vi "Update WayPt Angles.vi"(6 "Min R":dbl, 7 "Propagate":bool, 8 "Blends In":T1[](array[typedef]), 9 "Index":i32, 10 "Waypoints in":cluster{"x":dbl, "y":dbl, "th":dbl}[](array[cluster]), 11 "th":dbl) -> (1 "Blends Out":T1[](array[typedef]), 3 "Waypoints out":cluster{"x":dbl, "y":dbl, "th":dbl}[](array[cluster]))   [LabVIEW 2019]
uses:
  BlendType.ctl
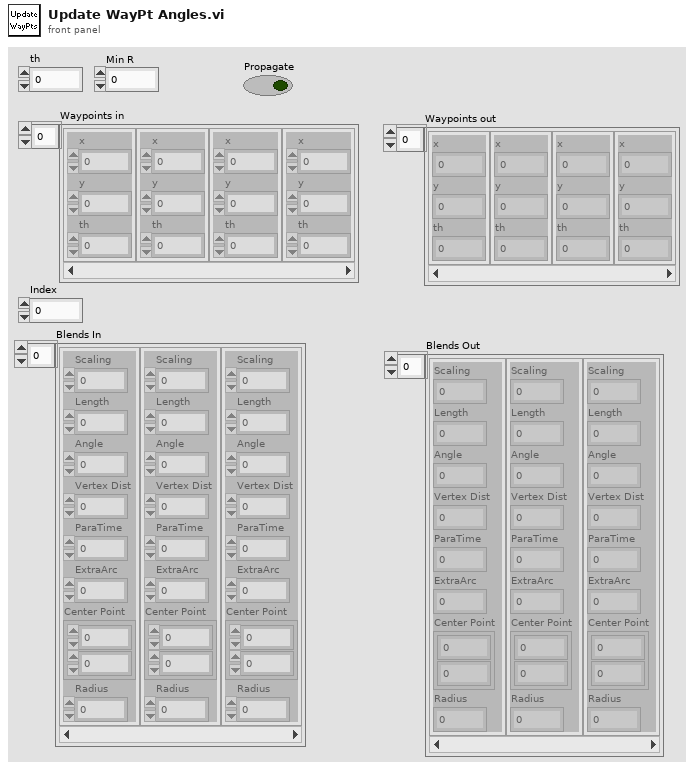
[diagram p1: front panel]
types:
  T1 = typedef "BlendType.ctl" = cluster{"Scaling":dbl, "Length":dbl, "Angle":dbl, "Vertex Dist":dbl, "ParaTime":dbl, "ExtraArc":dbl, "Center Point":cluster{dbl, dbl}, "Radius":dbl}
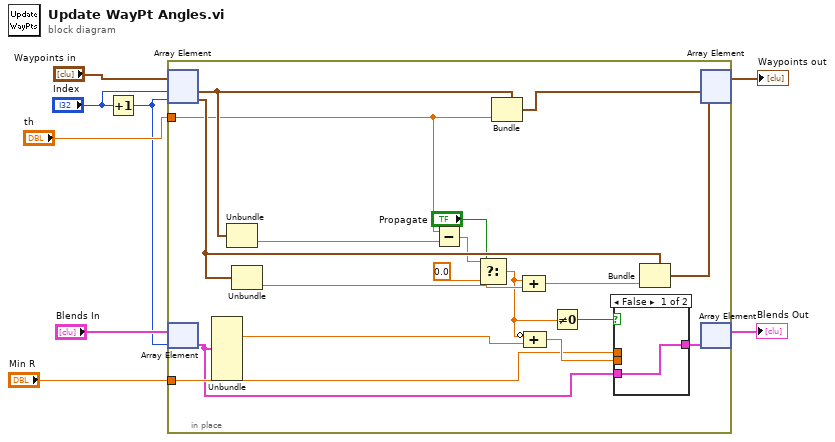
[diagram p0: block diagram]
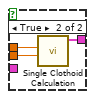
[diagram p2: hidden frame]
diagram:
  n1 = Increment(x="Index") -> (x+1=w1:i32)
  n2 = in-place {
    in-place-border: "th" -> [w14]
    in-place-border: "Min R" -> [w18]
    n3 = in-place-array #1("Waypoints in", "Index", w1) -> (w22:cluster{"x":dbl, "y":dbl, "th":dbl}, w25:cluster{"x":dbl, "y":dbl, "th":dbl})
    n4 = in-place-array #2("Blends In", w1) -> (w16:T1)
    n5 = Unbundle(w16) -> ("Angle"=w20:dbl)  [unwired: 7 out]
    n6 = Unbundle(w22) -> ("th"=w13:dbl)  [unwired: 2 out]
    n7 = Unbundle(w25) -> ("th"=w23:dbl)  [unwired: 2 out]
    n8 = Subtract(x=w14, y=w13) -> (x-y=w12:dbl)
    n9 = Select(t=w12, s="Propagate", f=0.0) -> (s? t:f=w10:dbl)
    n10 = Bundle(cluster=w22, "th"=w14) -> (w26:cluster{"x":dbl, "y":dbl, "th":dbl})  [unwired: 2 in]
    n11 = Compound Arithmetic op=ADD(w10, w23) -> (w21:dbl)
    n12 = Compound Arithmetic op=ADD(invert w10, w20) -> (w19:dbl)
    n13 = Not Equal To 0?(x=w10) -> (x != 0?=w15:bool)
    n14 = case shown="False" w15 {
      tunnel: w19 -> [_ w30]
      tunnel: w18 -> [_ w29]
      tunnel: [w27 w28] -> w17
      tunnel: w16 -> [w27 _]
      frame False {
      }
      frame True {
        n15 = call "Single Clothoid Calculation.vi"("Angle"=w30, "Min R"=w29) -> ("Zeroes out"=w28:T1)  [unwired: 9 in]
      }
    }
    n16 = Bundle(cluster=w25, "th"=w21) -> (w24:cluster{"x":dbl, "y":dbl, "th":dbl})  [unwired: 2 in]
    n17 = in-place-array #1(w26, w24) -> (→"Waypoints out":cluster{"x":dbl, "y":dbl, "th":dbl}[])  [unwired: 2 out]
    n18 = in-place-array #2(w17) -> (→"Blends Out":T1[])  [unwired: 1 out]
  }
